vi "citTemplate.queue.vi"(0 "ms timeout (250 ms)":i32=250, 2 "instance (0)":i32, 7 "event enum":variant, 11 "error in (no error)":errorcluster, 12 "iteration (-1)":i32=-1) -> (3 "notifierHandle out":T1, 4 "event out":u32, 8 "(flatten) data out":string, 14 "continue":bool, 15 "error out":errorcluster)   [LabVIEW 2016]
uses:
  citTemplate.notifierHandle.ctl
  citTemplate.notifierData.ctl
  citTemplate.eventQueue.ctl
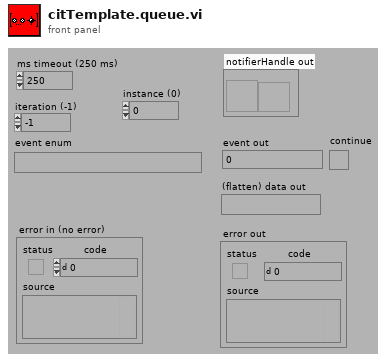
[diagram p1: front panel]
types:
  T1 = typedef "citTemplate.notifierHandle.ctl" = refnum<notifier>
  T2 = typedef "citTemplate.eventQueue.ctl" = enum16{"create queue", "get queue handle(s)", "destroy queue"}
  T3 = typedef "queueData.ctl" = cluster{"event index":u32, "(flatten) data in":string, "notifierHandle":T4}
  T4 = typedef "notifierHandle.ctl" = refnum<notifier>
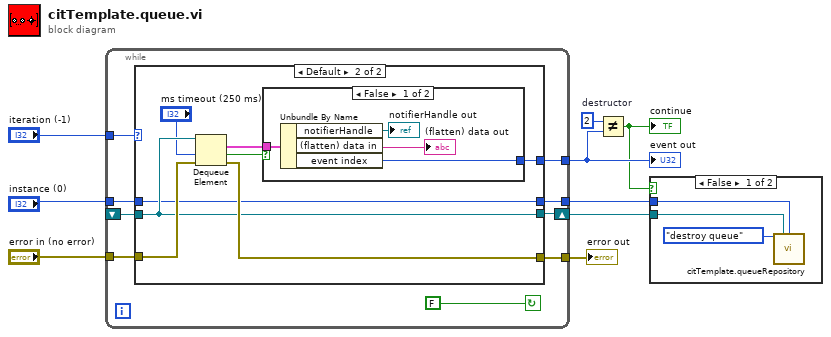
[diagram p0: block diagram]
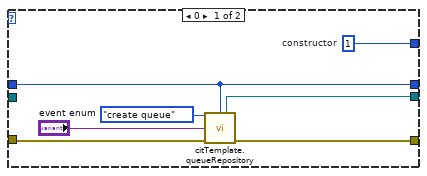
[diagram p3: hidden frame]
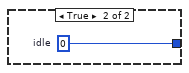
[diagram p4: hidden frame]
diagram:
  w6 = u32 2  # destructor
  n1 = while {
    tunnel: "error in (no error)" -> [w18]
    tunnel: [w12] -> w8
    tunnel: [w17] -> w5
    shift-right: [w13] -> w4
    shift-left: _ -> [w16]
    tunnel: "iteration (-1)" -> [w14]
    tunnel: [w11] -> w1
    tunnel: "instance (0)" -> [w10]
    stop <- FALSE continue-if-true
    n2 = case shown="Default" w14 {
      tunnel: w18 -> [w21 w31]
      tunnel: [w25 w33] -> w17
      tunnel: w16 -> [_ w28]
      tunnel: [w20 w28] -> w13
      tunnel: [w23 w29] -> w12
      tunnel: [w19 w26] -> w11
      tunnel: w10 -> [w19 w26]
      frame 0 {
        w25 = u32 1  # constructor
        n3 = call "citTemplate.queueRepository.vi"("mode (get queue handle)"=citTemplate.eventQueue."create queue" ("mode (write event)"), "instance (0)"=w19, "event in"="event enum", "error in (no error)"=w21) -> ("queue out"=w20:refnum<queue>, "error out"=w23:errorcluster)  [unwired: 3 in, 7 out]
      }
      frame Default {
        n4 = Dequeue Element(queue=w28, timeout in ms (-1)="ms timeout (250 ms)", error in (no error)=w31) -> (element=w32:T3, timed out?=w30:bool, error out=w29:errorcluster)  [unwired: 1 out]
        n5 = case shown="False" w30 {
          tunnel: [w36 w38] -> w33
          tunnel: w32 -> [w37 _]
          frame False {
            n6 = Unbundle By Name(w37) -> ("notifierHandle"=→"notifierHandle out":T4, "(flatten) data in"=→"(flatten) data out":string, "event index"=w36:u32)
          }
          frame True {
            w38 = u32 0  # idle
          }
        }
      }
    }
  }
  "event out" <- w5
  "error out" <- w8
  n7 = Not Equal?(x=w6, y=w5) -> (x != y?=w3:bool)
  "continue" <- w3
  n8 = case shown="False" w3 {
    tunnel: w4 -> [w40 _]
    tunnel: w1 -> [w39 _]
    frame False {
      n9 = call "citTemplate.queueRepository.vi"("mode (get queue handle)"=citTemplate.eventQueue."destroy queue" ("mode (write event)"), "queue in"=w40, "instance (0)"=w39) -> ()  [unwired: 4 in, 9 out]
    }
    frame True {
    }
  }
